vi "RobotLiftControl.vi"(11 "Robot Lift Command":T1) -> (3 "RobotLiftOutput out":T3)   [LabVIEW 2017]
uses:
  RobotLiftOutput.ctl
  RobotLiftCommand.ctl
  RunMode.ctl
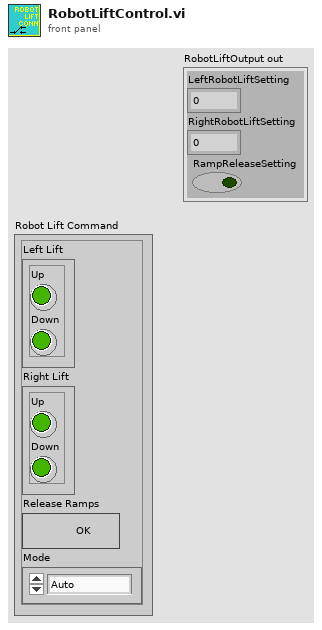
[diagram p1: front panel]
types:
  T1 = typedef "RobotLiftCommand.ctl" = cluster{"Left Lift":cluster{"Up":bool, "Down":bool}, "Right Lift":cluster{"Up":bool, "Down":bool}, "Release Ramps":bool, "Mode":T2}
  T2 = typedef "RunMode.ctl" = enum16{"Auto", "Teleop", "Disabled"}
  T3 = typedef "RobotLiftOutput.ctl" = cluster{"LeftRobotLiftSetting":dbl, "RightRobotLiftSetting":dbl, "RampReleaseSetting":bool}
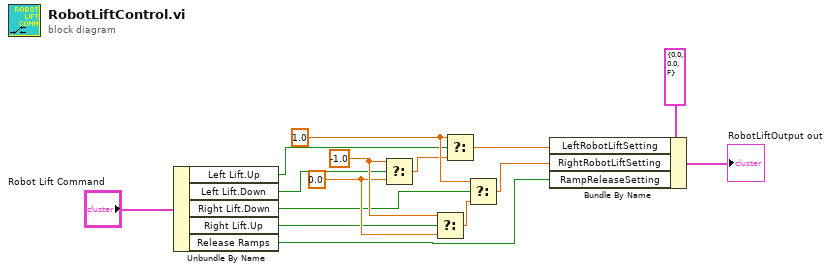
[diagram p0: block diagram]
diagram:
  w9 = 1.0
  w8 = -1.0
  w7 = 0.0
  n1 = Unbundle By Name("Robot Lift Command") -> ("Left Lift.Up"=w3:bool, "Left Lift.Down"=w4:bool, "Right Lift.Down"=w5:bool, "Right Lift.Up"=w6:bool, "Release Ramps"=w12:bool)
  n2 = Select(t=w8, s=w4, f=w7) -> (s? t:f=w2:dbl)
  n3 = Select(t=w8, s=w6, f=w7) -> (s? t:f=w1:dbl)
  n4 = Select(t=w9, s=w3, f=w2) -> (s? t:f=w14:dbl)
  n5 = Select(t=w9, s=w5, f=w1) -> (s? t:f=w13:dbl)
  n6 = Bundle By Name(cluster=T3 {"LeftRobotLiftSetting"=0.0, "RightRobotLiftSetting"=0.0, "RampReleaseSetting"=FALSE} ("RobotLiftOutput in"), "LeftRobotLiftSetting"=w14, "RightRobotLiftSetting"=w13, "RampReleaseSetting"=w12) -> (→"RobotLiftOutput out":T3)
